vi "Pose_Equals.vi"(9 "other POSE":T1, 11 "in POSE":T1) -> (3 "Equals":bool)   [LabVIEW 2019, in "Trajectory_Library.lvlib"]
doc: "Checks equality between this Pose2d and another Pose2d.\n\nParameters:\n - this Pose - This POSE2D data structure\n - other POSE - The other POSE2d data structure\n\nReturns: \n - Equals - Value will be TRUE if both POSEs are the same"
uses:
  Trajectory_Library.lvlib
  POSE2D.ctl
  TRANSLATION2D.ctl
  ROTATION2D.ctl
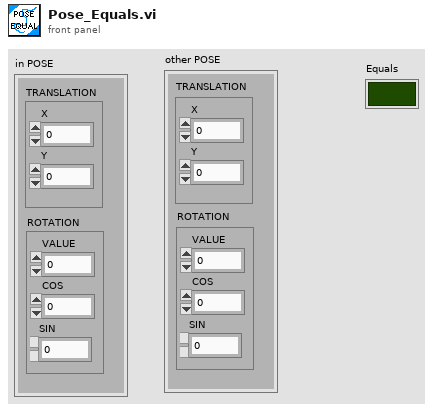
[diagram p1: front panel]
types:
  T1 = typedef "Trajectory_Library.lvlib/POSE2D.ctl" = cluster{"TRANSLATION":T2, "ROTATION":T3}
  T2 = typedef "Trajectory_Library.lvlib/TRANSLATION2D.ctl" = cluster{"X":dbl, "Y":dbl}
  T3 = typedef "Trajectory_Library.lvlib/ROTATION2D.ctl" = cluster{"VALUE":dbl, "COS":dbl, "SIN":dbl}
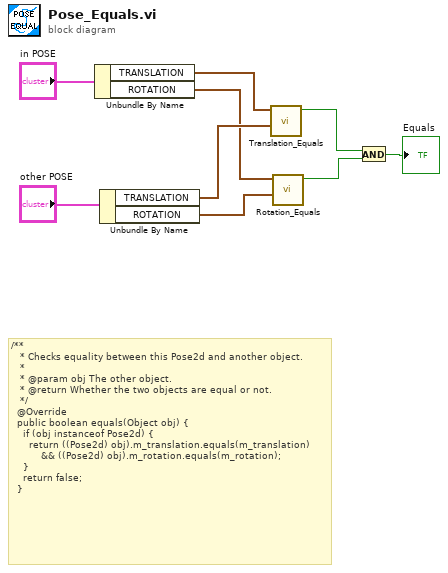
[diagram p0: block diagram]
diagram:
  # "/**\n   * Checks equality between this Pose2d and another object.\n   *\n   * @param obj The other object.\n   * @return Whether the two objects are equal or not.\n   */\n  @Override\n  public boolean equals(Object obj) {\n    if (obj instanceof Pose2d) {\n      return ((Pose2d) obj).m_translation.equals(m_translation)\n          && ((Pose2d) obj).m_rotation.equals(m_rotation);\n    }\n    return false;\n  }"
  n1 = Unbundle By Name("in POSE") -> ("TRANSLATION"=w6:T2, "ROTATION"=w4:T3)
  n2 = Unbundle By Name("other POSE") -> ("TRANSLATION"=w5:T2, "ROTATION"=w3:T3)
  n3 = call "Translation_Equals.vi"("other Translation"=w5, "In Translation"=w6) -> ("Equals"=w2:bool)  [unwired: 9 in]
  n4 = call "Rotation_Equals.vi"("other ROTATION"=w3, "in ROTATION"=w4) -> ("Equals"=w1:bool)  [unwired: 9 in]
  n5 = And(x=w2, y=w1) -> (x .and. y?=→"Equals":bool)
